vi "PassObserverSkill.vi"(8 "error in (no error)":errorcluster, 9 "Game in":refnum<class "Game.lvclass">, 10 "Robot":refnum<class "Robot.lvclass">, 11 "PassObserverSkill in":refnum<class "PassObserverSkill.lvclass">) -> (0 "error out":errorcluster, 1 "Boolean":bool, 2 "Robot":refnum<class "Robot.lvclass">, 3 "PassObserverSkill out":refnum<class "PassObserverSkill.lvclass">)   [LabVIEW 2023, in "PassObserverSkill.lvclass"]
uses:
  PassObserverSkill.lvclass
  Robot_class/Robot.lvclass
  Game_class/Game.lvclass
  Utilities_class/Utilities.lvclass
  Robot_class/tactics.ctl
  Object_class/Object.lvclass/Object.ctl
  Game_class/Game.lvclass/Game.ctl
  Team_class/Team.lvclass/Team.ctl
  Parameters_class/Parameters.lvclass/Parameters.ctl
  Robot_class/roles.ctl
  Robot_class/Robot.lvclass/Robot.ctl
  Game_class/Read OffensiveTeam.vi
  Game_class/Read FieldRef.vi
  Game_class/Read BallRef.vi
  Game_class/Read Parameters.lvclass.vi
  Parameters_class/Read AttakingOurselves.vi
  Object_class/Read x.vi
  Object_class/Read y.vi
  Team_class/Read OffensivePlay.vi
  Team_class/Read RobotRef.vi
  Robot_class/Read tactic.vi
  Robot_class/Write dest_x.vi
  Robot_class/Write dest_y.vi
  Robot_class/Write dest_orientation.vi
  Ball_class/Ball.lvclass
  Ally_class/Ally.lvclass
  Field_class/Field.lvclass
  Parameters_class/Parameters.lvclass
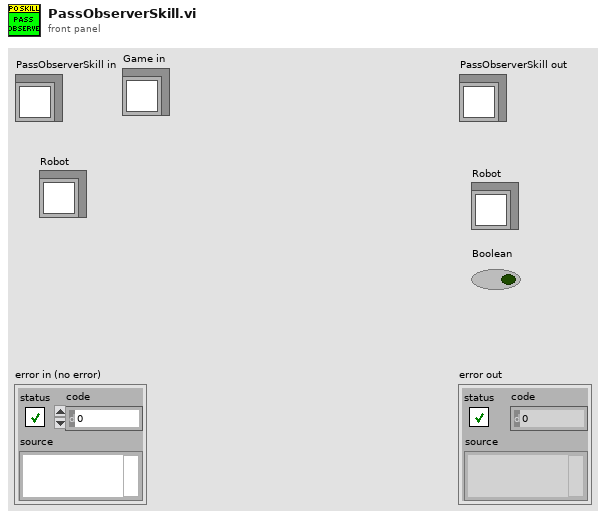
[diagram p1: front panel]
types:
  T1 = typedef "tactics.ctl" = enum16{"ReceivePassInFuturePoint", "Roller", "PrepareRollToPassRollerGoTo", "PrepareRollToPassReceiverGoTo", "WaitRoll", "PositionToRoll", "PenaltyAttacker", "PassObserver", "PenaltyDefense", "TableReceiverTactic", "Test", "DefendGoal", "Marker", "FollowAttacker", "DefendArea", "Shoot", "AttackerAimGoal", "AttackerBallOutOfField", "AttackerBlock", "AttackerStop", "Duelist", "Halt", "ZigZag", "GoTo", "Timeout", "KickToPassReceiver", "PositionToReceivePass", "DefendAreaVSS", "DefendGoalVSS", "KickVSS", "AttackVSS", "DispBallVSS", "PenaltyAttackVSS", "WaitPass"}
  T2 = typedef "roles.ctl" = enum16{"BallChallengerAttackerVSS", "NormalAttackerVSS", "AttackerAimGoalVSS", "DefenderAreaVSS", "KeeperVSS", "Tabler", "TableFinalizer", "PrepareRollToPassRoller", "PrepareRollToPassReceiver", "SimplePassRoll", "SimplePassRollReceiver", "PenaltyDefense", "PreparePassReceiver 2", "PreparePassReceiver 1", "PassObserver", "Timeout", "Goto", "ZigZag", "None", "BallOutOfField", "DefenderArea", "Duelist", "AttackerStop", "FollowAttacker", "KeeperRole", "KickPenalty", "AttackerAimGoal", "AttackerBlock", "Marker", "Halt", "Shoot", "PassKicker", "PassReceiver", "TestRole", "PenaltyAttacker"}
  T3 = typedef "OffensivePlay.ctl" = enum16{"TableWithStriker", "TableWith2ndStrikerPlay", "PrepareDoublePass", "PrepareRollToPass", "SimplePass", "PreparePass", "PassToStriker", "BallOutOfField", "PassTo2ndStriker", "StopOffensive", "Prepare Penalty Enemy", "EnemyPossessionAtEnemyField", "EnemyPossesionAtOurField", "TestPlay", "PreparePenaltyAlly", "KickPenaltyAlly", "PrepareKickoffAlly", "PrepareKickoffEnemy", "IndirectEnemy", "DirectEnemy", "NormalGame", "DirectKick", "Pass", "Halt", "Timeout", "PassPlay", "PenaltyEnemy"}
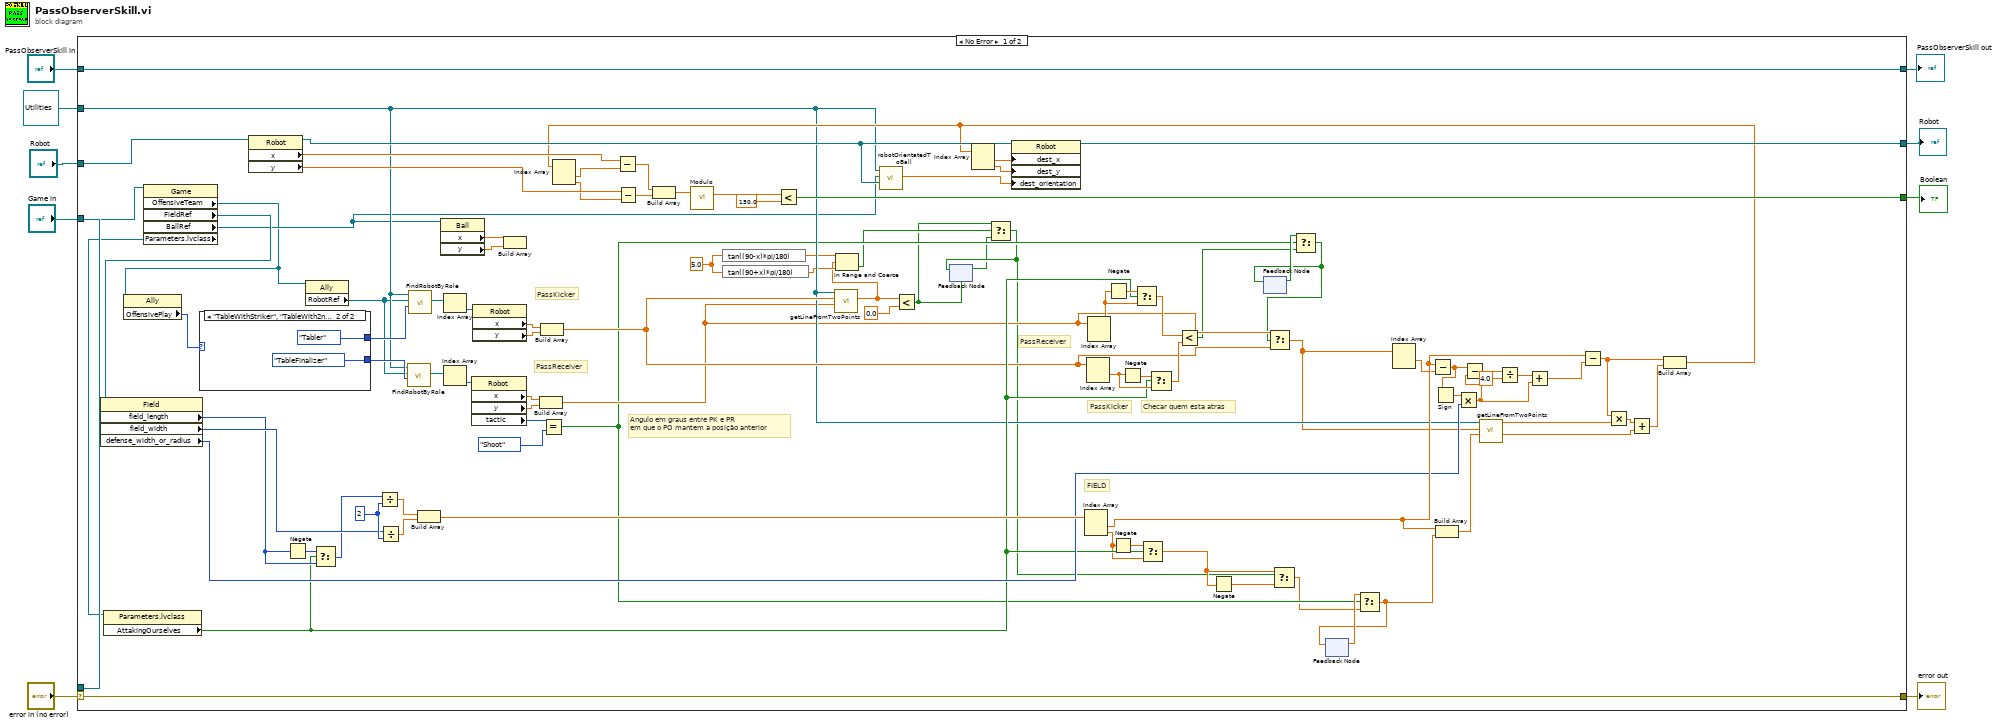
[diagram p0: block diagram]
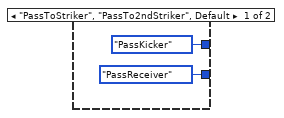
[diagram p2: hidden frame]
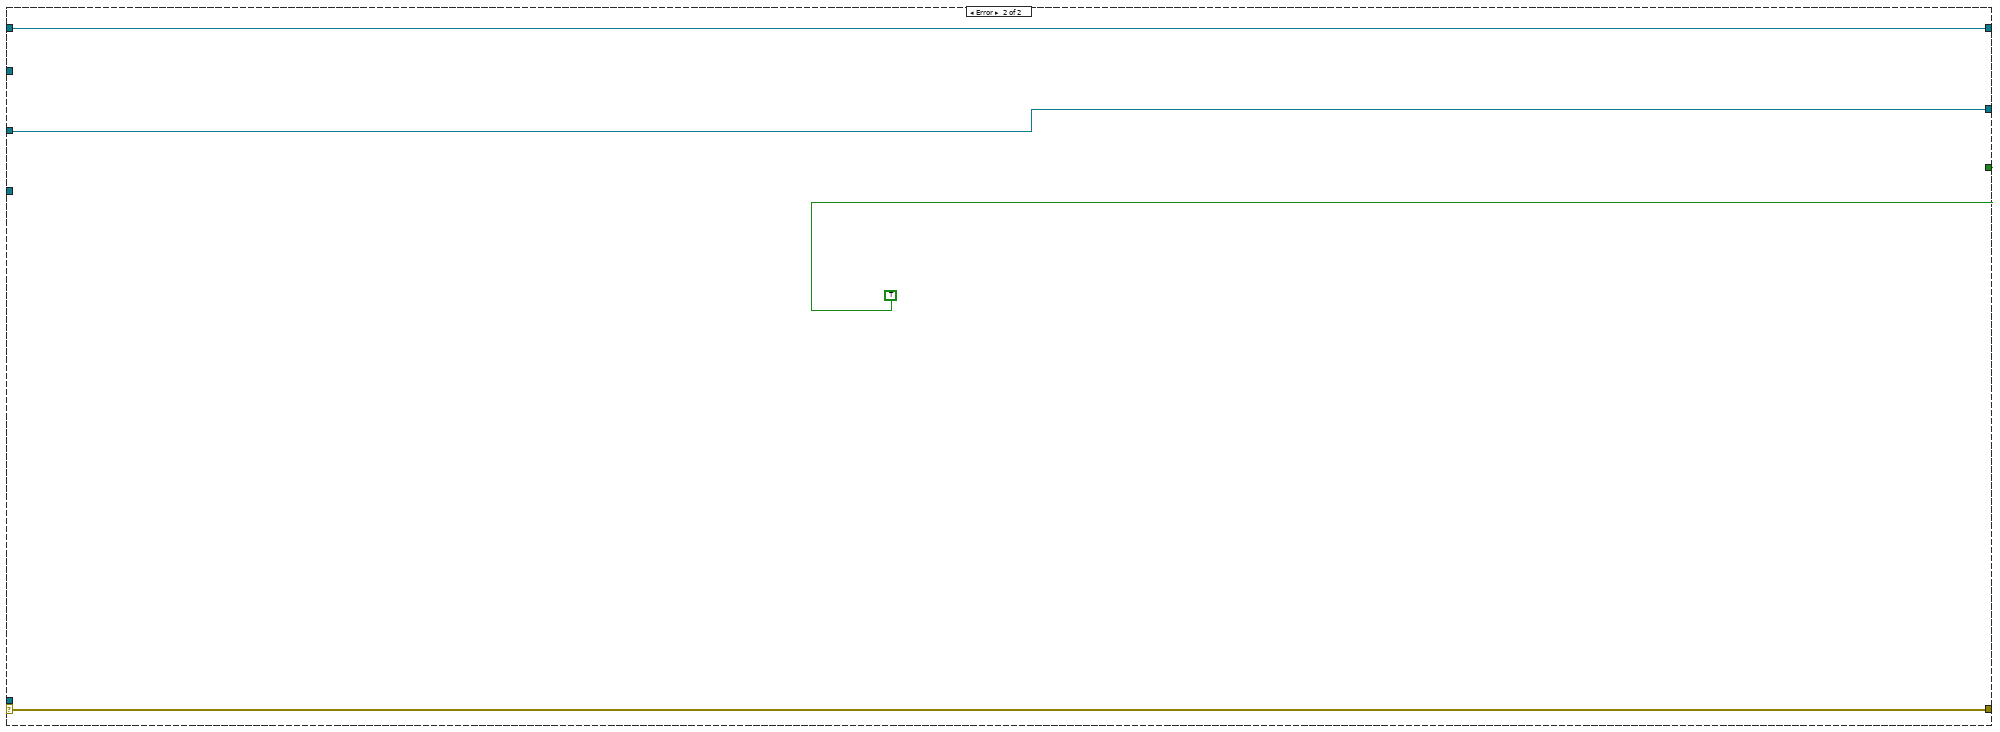
[diagram p3: hidden frame]
diagram:
  n1 = case shown="No Error" "error in (no error)" {
    selector: "error in (no error)" -> [w86 w112]
    tunnel: [w86 w112] -> w8
    tunnel: [w104 w111] -> w6
    tunnel: "PassObserverSkill in" -> [w104 w111]
    tunnel: "Robot" -> [w85 w110]
    tunnel: [w103 w110] -> w4
    tunnel: [w97 TRUE] -> w2
    tunnel: "Game in" -> [w96 _]
    tunnel: "Game in" -> [_ _]
    tunnel: refnum<class "Utilities.lvclass"> refnum ("Utilities in") -> [w33 _]
    frame No Error {
      w19 = 5.0
      w94 = 2
      # "Angulo em graus entre PK e PR \nem que o PO mantem a posição anterior"
      # "PassReceiver"
      # "Checar quem esta atras"
      # "PassReceiver"
      # "FIELD"
      # "PassKicker"
      # "PassKicker"
      n2 = property class="Game"(reference=w96) -> ("OffensiveTeam"=w11:refnum<class "Ally.lvclass">, "FieldRef"=w95:refnum<class "Field.lvclass">, "BallRef"=w12:refnum<class "Ball.lvclass">, "Parameters.lvclass"=w64:refnum<class "Parameters.lvclass">)  [unwired: 1 in, 2 out]
      n3 = property class="Field"(reference=w95) -> ("field_length"=w61:i32, "field_width"=w90:i32, "defense_width_or_radius"=w52:i32)  [unwired: 1 in, 2 out]
      n4 = property class="Parameters.lvclass"(reference=w64) -> ("AttakingOurselves"=w49:bool)  [unwired: 1 in, 2 out]
      n5 = property class="Ally"(reference=w11) -> ("OffensivePlay"=w10:T3)  [unwired: 1 in, 2 out]
      n6 = case shown="\"TableWithStriker\", \"TableWith2ndStrikerPlay\"" w10 {
        tunnel: [roles."PassKicker" ("y") roles."Tabler" ("y")] -> w44
        tunnel: [roles."PassReceiver" ("y") roles."TableFinalizer" ("y")] -> w38
        frame "PassToStriker", "PassTo2ndStriker", Default {
        }
        frame "TableWithStriker", "TableWith2ndStrikerPlay" {
        }
      }
      n7 = property class="Robot"(reference=w85) -> (reference out=w87:refnum<class "Robot.lvclass">, "x"=w93:dbl, "y"=w92:dbl)  [unwired: 1 in, 1 out]
      n8 = Negate(x=w61) -> (-x=w62:i32)
      n9 = property class="Ally"(reference=w11) -> ("RobotRef"=w32:refnum<class "Robot.lvclass">[])  [unwired: 1 in, 2 out]
      n10 = Select(t=w62, s=w49, f=w61) -> (s? t:f=w60:i32)
      n11 = Divide(x=w60, y=w94) -> (x/y=w78:dbl)
      n12 = Divide(x=w90, y=w94) -> (x/y=w91:dbl)
      n13 = call "FindRobotByRole.vi"("role"=w38, "RobotRef"=w32, "Utilities in"=w33) -> ("Robots"=w37:refnum<class "Robot.lvclass">[])  [unwired: 6 in, 2 out]
      n14 = call "FindRobotByRole.vi"("role"=w44, "RobotRef"=w32, "Utilities in"=w33) -> ("Robots"=w43:refnum<class "Robot.lvclass">[])  [unwired: 6 in, 2 out]
      n15 = Build Array(w78, w91) -> (w66:dbl[])
      n16 = property class="Ball"(reference=w12) -> ("x"=w80:dbl, "y"=w79:dbl)  [unwired: 1 in, 2 out]
      n17 = Index Array(array=w37) -> (element=w36:refnum<class "Robot.lvclass">)  [unwired: 1 in]
      n18 = Index Array(array=w43) -> (element=w42:refnum<class "Robot.lvclass">)  [unwired: 1 in]
      n19 = property class="Robot"(reference=w36) -> ("x"=w35:dbl, "y"=w34:dbl, "tactic"=w29:T1)  [unwired: 1 in, 2 out]
      n20 = property class="Robot"(reference=w42) -> ("x"=w41:dbl, "y"=w40:dbl)  [unwired: 1 in, 2 out]
      n21 = Build Array(w80, w79) -> ()  [unwired: 1 out]
      n22 = Build Array(w35, w34) -> (w31:dbl[])
      n23 = Build Array(w41, w40) -> (w39:dbl[])
      n24 = Equal?(x=w29, y=tactics."Shoot" ("tactic")) -> (x = y?=w26:bool)
      n25 = expression code="tan((90-x)*pi/180)"(w19) -> (w17:dbl)
      n26 = expression code="tan((90+x)*pi/180)"(w19) -> (w18:dbl)
      n27 = call "getLineFromTwoPoints.vi"("Point 2"=w31, "Point 1"=w39, "Utilities in"=w33) -> ("angular coef"=w16:dbl)  [unwired: 4 in, 4 out]
      n28 = In Range and Coerce(upper limit=w17, x=w16, lower limit=w18) -> (In Range?=w15:bool)  [unwired: 1 out]
      n29 = call "robotOrientatedToBall.vi"("Robot"=w87, "BallRef"=w12, "Utilities in"=w33) -> ("Orientation"=w88:dbl)  [unwired: 6 in, 2 out]
      n30 = Less?(x=w16, y=0.0) -> (x < y?=w14:bool)
      n31 = feedback #1(w14) -> (w13:bool)
      n32 = Select(t=w14, s=w15, f=w13) -> (s? t:f=w20:bool)
      n33 = feedback-in #1(w20) -> ()
      n34 = Index Array(array=w66) -> (element #1=w73:dbl, element #2=w46:dbl)  [unwired: 2 in]
      n35 = Index Array(array=w39) -> (element #1=w55:dbl)  [unwired: 2 in, 1 out]
      n36 = Index Array(array=w31) -> (element #1=w57:dbl)  [unwired: 2 in, 1 out]
      n37 = Negate(x=w57) -> (-x=w59:dbl)
      n38 = Negate(x=w46) -> (-x=w47:dbl)
      n39 = Negate(x=w55) -> (-x=w56:dbl)
      n40 = Select(t=w59, s=w49, f=w57) -> (s? t:f=w58:dbl)
      n41 = Select(t=w47, s=w49, f=w46) -> (s? t:f=w48:dbl)
      n42 = Select(t=w56, s=w49, f=w55) -> (s? t:f=w45:dbl)
      n43 = Less?(x=w58, y=w45) -> (x < y?=w22:bool)
      n44 = Negate(x=w48) -> (-x=w63:dbl)
      n45 = feedback #2() -> (w28:bool)  [unwired: 1 in]
      n46 = Select(t=w48, s=w20, f=w63) -> (s? t:f=w24:dbl)
      n47 = Select(t=w28, s=w26, f=w22) -> (s? t:f=w21:bool)
      n48 = feedback-in #2(w21) -> ()
      n49 = Select(t=w31, s=w21, f=w39) -> (s? t:f=w23:dbl[])
      n50 = feedback #3() -> (w27:dbl)  [unwired: 1 in]
      n51 = Select(t=w27, s=w26, f=w24) -> (s? t:f=w25:dbl)
      n52 = feedback-in #3(w25) -> ()
      n53 = Index Array(array=w23) -> (element #1=w67:dbl)  [unwired: 2 in, 1 out]
      n54 = Subtract(x=w73, y=w67) -> (x-y=w54:dbl)
      n55 = Sign(1:w54) -> (0:w53:dbl)
      n56 = Build Array(w73, w25) -> (w77:dbl[])
      n57 = Multiply(x=w53, y=w52) -> (x*y=w51:dbl)
      n58 = Subtract(x=w54, y=w51) -> (x-y=w76:dbl)
      n59 = call "getLineFromTwoPoints.vi"("Point 2"=w77, "Point 1"=w23, "Utilities in"=w33) -> ("linear coef"=w70:dbl, "angular coef"=w72:dbl)  [unwired: 4 in, 3 out]
      n60 = Divide(x=w76, y=4.0) -> (x/y=w74:dbl)
      n61 = Add(x=w74, y=w51) -> (x+y=w50:dbl)
      n62 = Subtract(x=w73, y=w50) -> (x-y=w69:dbl)
      n63 = Multiply(x=w69, y=w72) -> (x*y=w71:dbl)
      n64 = Add(x=w71, y=w70) -> (x+y=w68:dbl)
      n65 = Build Array(w69, w68) -> (w65:dbl[])
      n66 = Index Array(array=w65) -> (element #1=w82:dbl, element #2=w81:dbl)  [unwired: 2 in]
      n67 = Subtract(x=w93, y=w82) -> (x-y=w102:dbl)
      n68 = Subtract(x=w92, y=w81) -> (x-y=w101:dbl)
      n69 = Build Array(w102, w101) -> (w100:dbl[])
      n70 = call "Modulo.vi"("2D vector"=w100) -> ("Modulo"=w98:dbl)  [unwired: 10 in]
      n71 = Less?(x=w98, y=150.0) -> (x < y?=w97:bool)
      n72 = Index Array(array=w65) -> (element #1=w84:dbl, element #2=w83:dbl)  [unwired: 2 in]
      n73 = property class="Robot"(reference=w87, "dest_x"=w84, "dest_y"=w83, "dest_orientation"=w88) -> (reference out=w103:refnum<class "Robot.lvclass">)  [unwired: 1 in, 1 out]
    }
    frame Error {
    }
  }
  "error out" <- w8
  "PassObserverSkill out" <- w6
  "Robot" <- w4
  "Boolean" <- w2
